vi "Scope_5782_PID_test.vi"() -> ()   [LabVIEW 2013]
uses:
  <vilib>/userdefined/High Color/nirio_resource_hc.ctl
  FPGA/DataMode.ctl
  <vilib>/Analysis/4window.llb/windowTd.ctl
  Host/Scope/controls/power_spectrum_unit.ctl
  Host/Scope5782/Scope/controls/5782_trigger_type.ctl
  Host/Scope/controls/Data_calc_mode.ctl
  Host/Scope/controls/Data_display_mode.ctl
  Host/Scope/controls/Graph_references.ctl
  Host/Scope/controls/graph_controls.ctl
  Host/Scope/controls/Channel_select.ctl
  Host/Scope5782/Config/FPGAref_5782.ctl
  Host/Scope/controls/ScopeMode.ctl
  <vilib>/FPGAPlugInAG/PXIe-7975R/niLvFpga_Open_PXIe-7975R.vi
  <vilib>/rvi/interface/common/dynamic/niFpgaDynamicAddResources.vi
  <vilib>/rvi/interface/common/niFpgaWaitOnOcc.vi
  <vilib>/Utility/error.llb/Error Cluster From Error Code.vi
  <vilib>/rvi/errors/niLvFpgaAdjustHostInterfaceError.vi
  <vilib>/FPGAPlugInAG/Dynamic/niLvFpga_Close_Dynamic.vi
  <vilib>/rvi/interface/nirviOpenFPGA/nirviOpenFPGA.xnode
  FPGA Bitfiles/mixer_FPGATarget2_FPGAmain5782PIDt_FQeTUQzgJng.lvbitx
  <vilib>/rvi/interface/nirviReadWriteControl/nirviReadWriteControl.xnode
  <vilib>/rvi/interface/nirviCloseFPGA/nirviCloseFPGA.xnode
  Host/Utilities/Ticker/Ticker.lvclass
  NiFpgaLv.dll
  <vilib>/rvi/interface/Simulation/niFpgaSimulationCallBeginRW.vi
  <vilib>/Analysis/NI_AALPro.lvlib
panel:
  in  "Kp":fxp<+/-,32,4>
  in  "Kd/T":fxp<+/-,32,4>
  in  "Ki*T":fxp<+/-,32,4>
  in  "Feedback":bool
  in  "b":fxp<+/-,16,2>
  in  "a":fxp<+/-,16,2>
  in  "Fequency [kHz]":dbl format="%#_8g"
  in  "#bins":i32=1 min=1 max=16
  in  "ch1 DC offset":i16 caption="DC offset\nChannel 1"
  in  "ch0 DC offset":i16 caption="DC offset\nChannel 0"
  in  "Output delay delta":dbl(slide) scale=0.0..6.0
  in  "Output delay":dbl(slide) scale=0.0..6.0
  in  "Chart length":i32=200000
  in  "Trigmode":enum32{"Triggered", "Continuous"}(radio)
  in  "Refence for phase":T1
  in  "Graph_refs":T2
  out "Lower chart":dbl[][](graph)
  out "Upper chart":dbl[][](graph)
  out "Lower graph":i16[][](graph)
  in  "Buffer":T4
  in  "Display":T5
  in  "Output mixer fequency [MHz]":dbl
  in  "Trigger":T6
  in  "Ch1 Q":bool
  in  "Ch1 I":bool
  in  "Ch0 Q":bool
  in  "Ch0 I":bool
  in  "Ch1":bool
  in  "Ch0":bool
  out "stop 2":bool
  in  "Zoom freq X":bool
  in  "Zoom freq Y":bool
  in  "Zoom time Y":bool
  in  "Zoom time X":bool
  in  "Unit":T7
  in  "Window":T8=1 items=["Rectangle"=0, "Hanning"=1, "Hamming"=2, "Blackman-Harris"=3, "Exact Blackman"=4, "Blackman"=5, "Flat Top"=6, "4 Term B-Harris "=7, "7 Term B-Harris"=8, "Low Sidelobe"=9, "Blackman Nuttall"=11, "Triangle"=30, "Bartlett-Hanning"=31, "Bohman"=32, "Parzen"=33, "Welch"=34, "Kaiser"=60, "Dolph-Chebyshev"=61, "Gaussian"=62]
  in  "Samples per 5782 record":i32
  in  "Phase offset (deg)":dbl
  in  "Fequency [MHz]":dbl format="%#_8g"
  in  "Mode":T9
  in  "Mixer freq [MHz]":dbl
  out "freqdata":cluster{"f0":dbl, "df":dbl, "magnitude":dbl[]}[](graph)
  out "Upper graph":i16[][](graph)
  in  "Rumode":bool
  in  "Singleshot":bool
  out "error IO":errorcluster
  in  "stop":bool
  in  "resource name":T10="RIO0"
  out "Clocking Option Configured?":bool
  out "Configured?":bool
  # "FPGA setup"
  # "ADU"
  # "ADU"
  # "Output delay"
  # "ns"
  # "Auto Zoom"
  # "Output delay delta"
  # "ps"
  # "5782"
  # "Amplitude modulation"
  # "Simulated data"
  # "FFT"
  # "Auto Zoom"
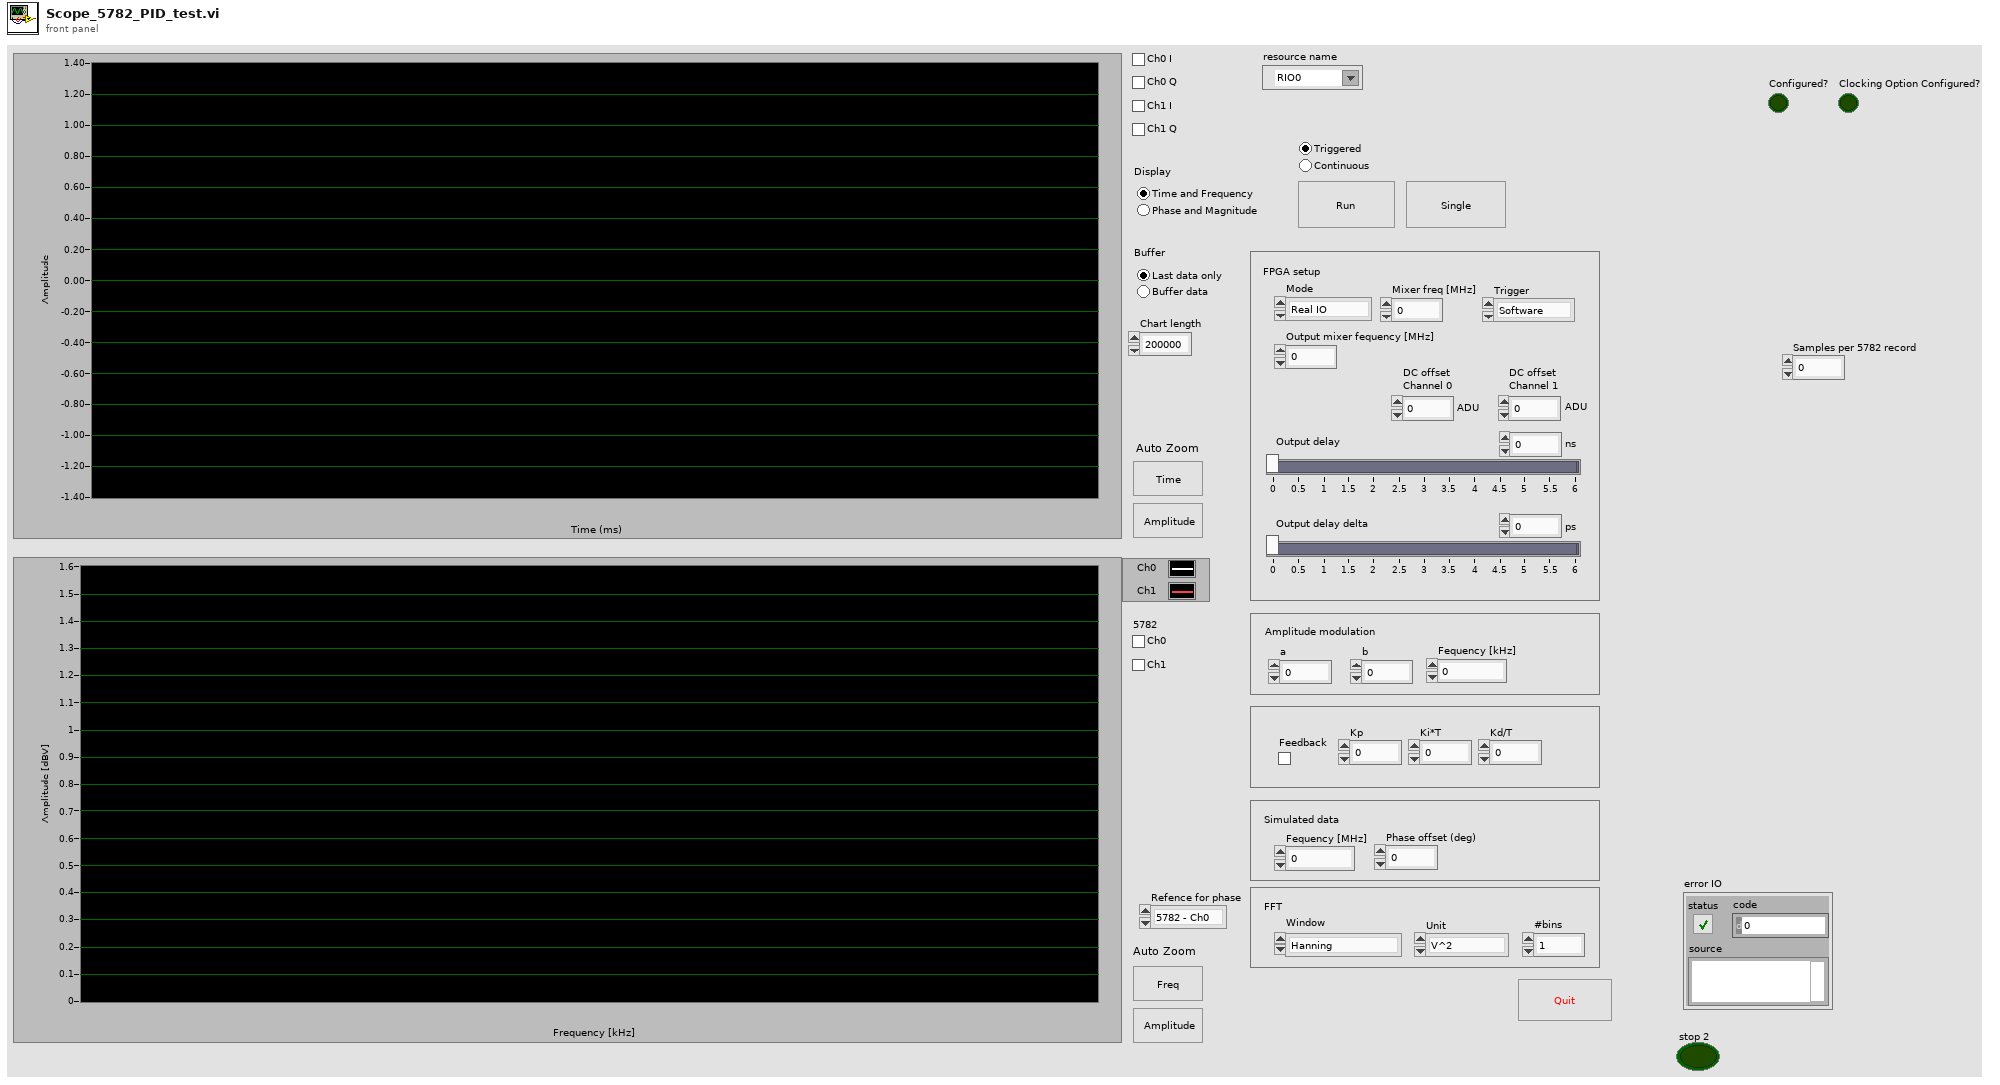
[diagram p1: front panel]
types:
  T1 = typedef "Channel_select.ctl" = enum16{"5782 - Ch0", "5782 - Ch1"}
  T2 = typedef "Graph_references.ctl" = cluster{"upper":T3, "lower":T3, "Freq graph":refnum<vi>}
  T3 = typedef "graph_controls.ctl" = cluster{"Graph":refnum<vi>, "Time btn":refnum<vi>, "Amplitude btn":refnum<vi>, "Chart":refnum<vi>}
  T4 = typedef "Data_display_mode.ctl" = enum32{"Last data only", "Buffer data"}
  T5 = typedef "Data_calc_mode.ctl" = enum32{"Time and Frequency", "Phase and Magnitude"}
  T6 = typedef "5782_trigger_type.ctl" = enum16{"Software", "Trigger input"}
  T7 = typedef "power_spectrum_unit.ctl" = enum16{"V^2", "V", "dBV"}
  T8 = typedef "NI_AALPro.lvlib/windowTd.ctl" = u32
  T9 = typedef "DataMode.ctl" = enum16{"Real IO", "Simulated"}
  T10 = typedef "nirio_resource_hc.ctl" = tag
  T11 = typedef "FPGAref_5782.ctl" = refnum<k20>
  T12 = enum8{"Internal Clock PLL Off", "Internal Clock PLL On (REF IN)", "External Clock (CLK_IN)", "Internal Clock PLL On (IoModSyncClk)"}
  T13 = typedef "scope_params_5782.ctl" = cluster{"scope mode":T14, "ticker":refnum<class "Ticker.lvclass">, "samples per record":i32, "FPGA ref":T11, "data mode":T9, "5782 Trigger":T6, "Chart length":i32}
  T14 = typedef "ScopeMode.ctl" = enum16{"Stopped", "Single", "Running", "Continuous"}
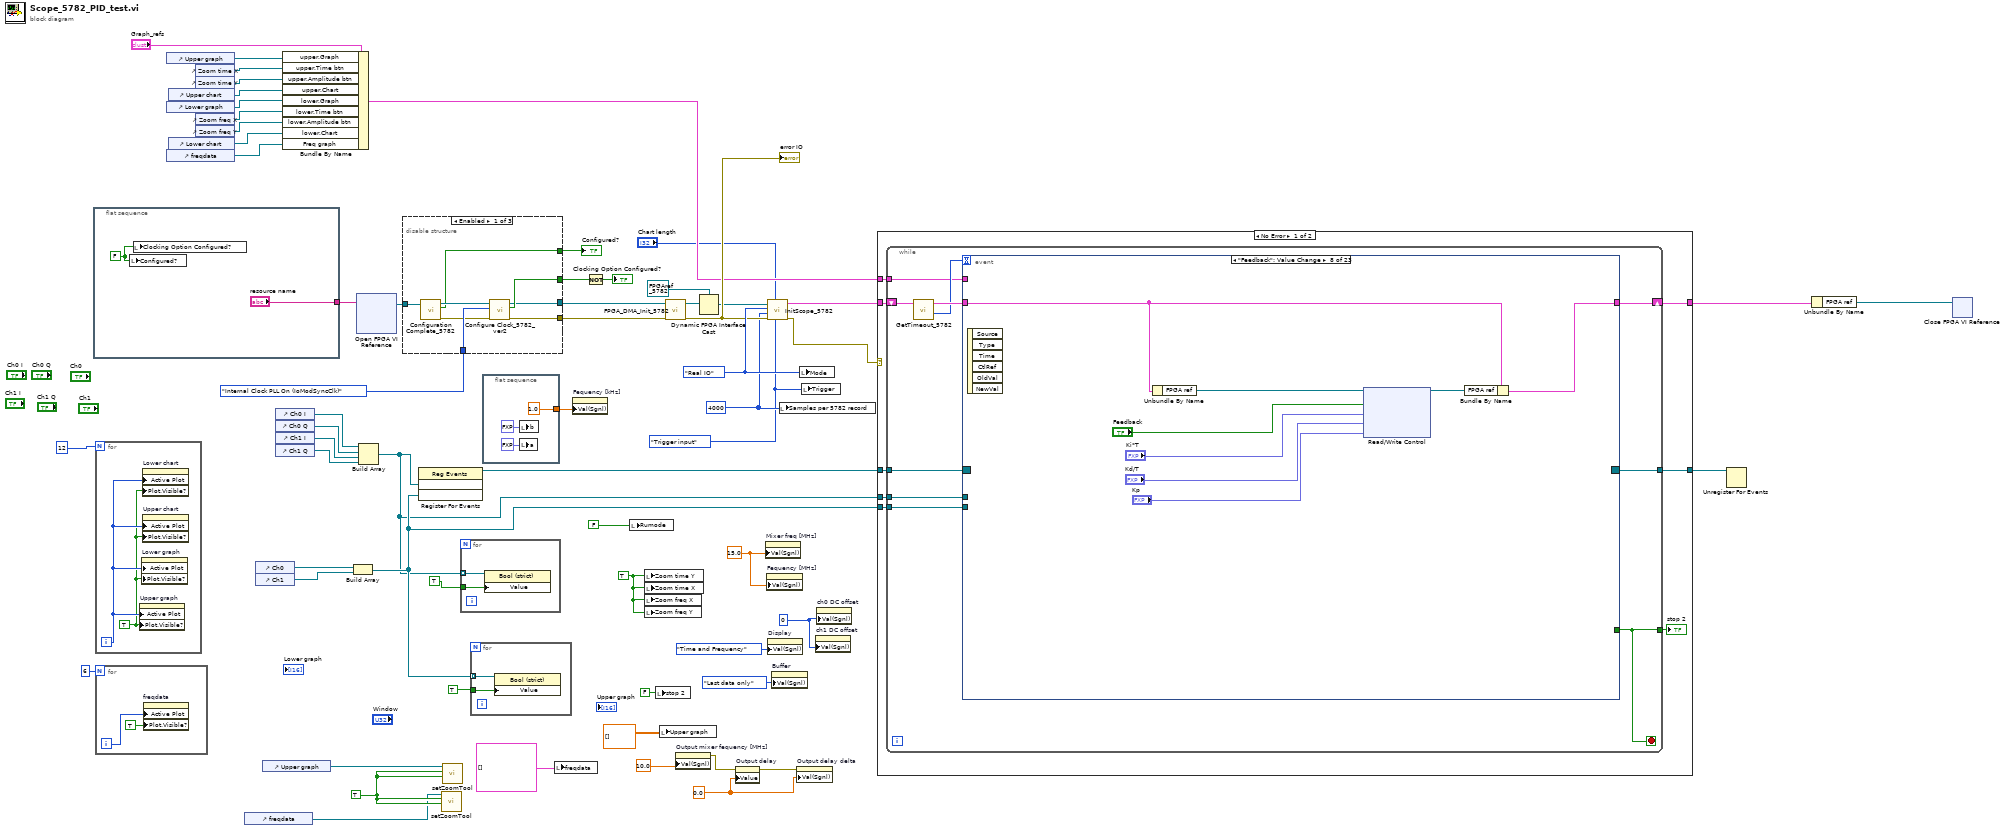
[diagram p0: block diagram]
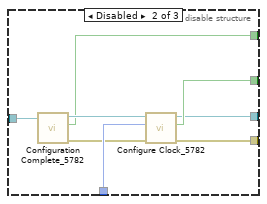
[diagram p2: hidden frame]
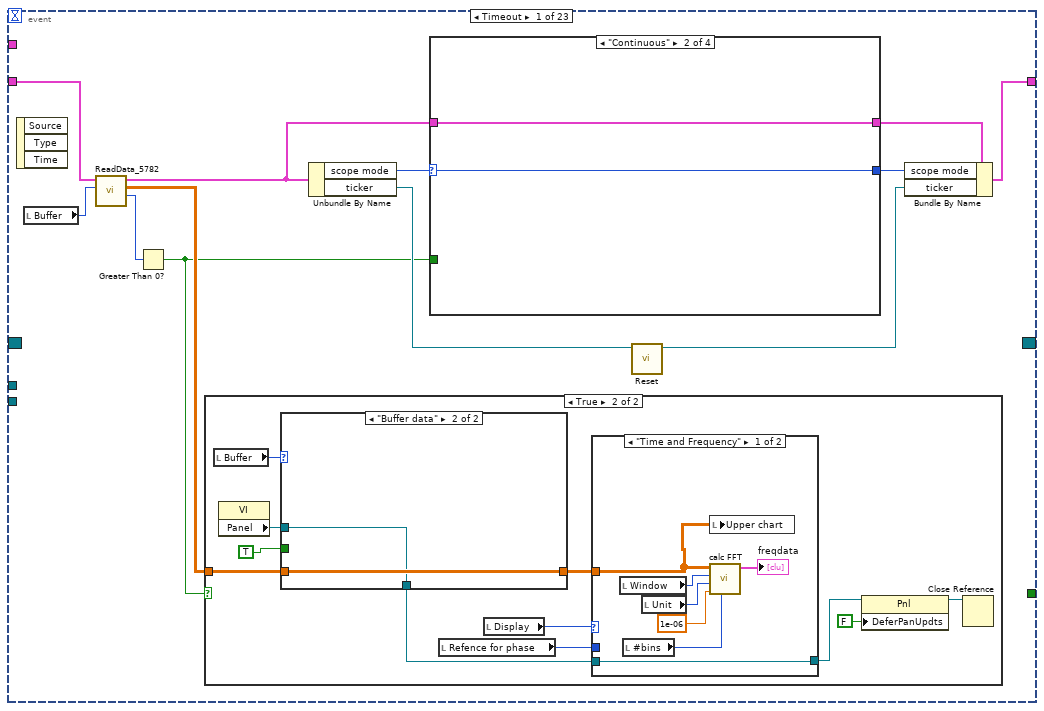
[diagram p4: hidden frame]
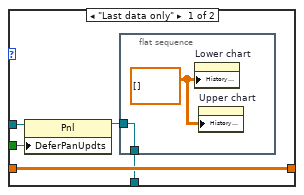
[diagram p6: hidden frame]
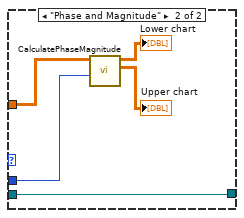
[diagram p7: hidden frame]
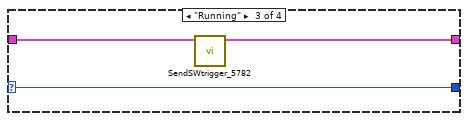
[diagram p9: hidden frame]
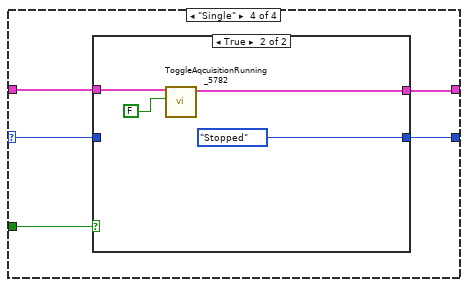
[diagram p10: hidden frame]
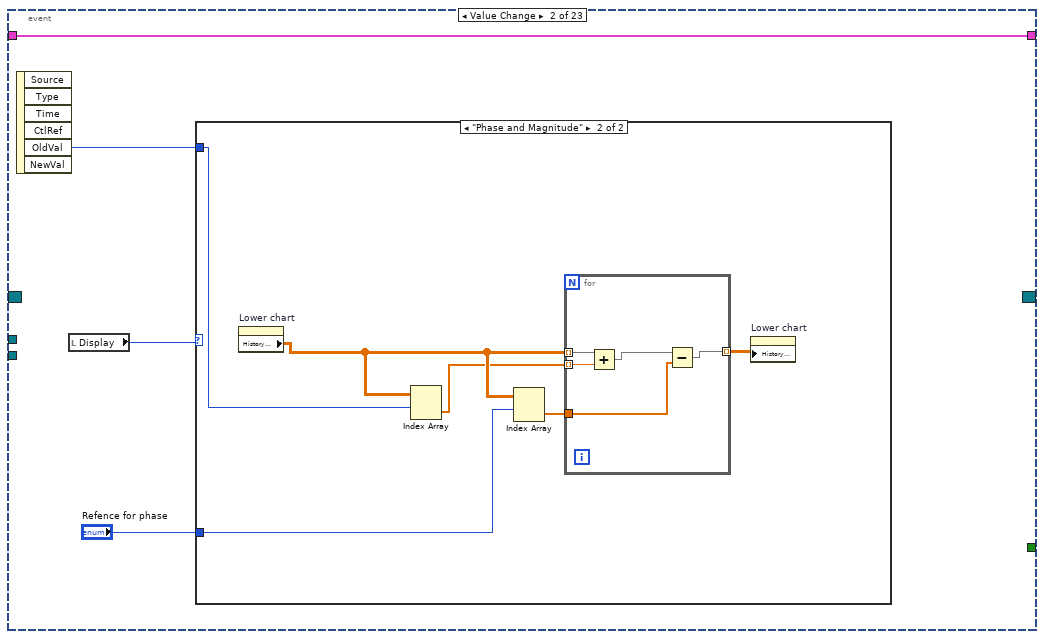
[diagram p12: hidden frame]
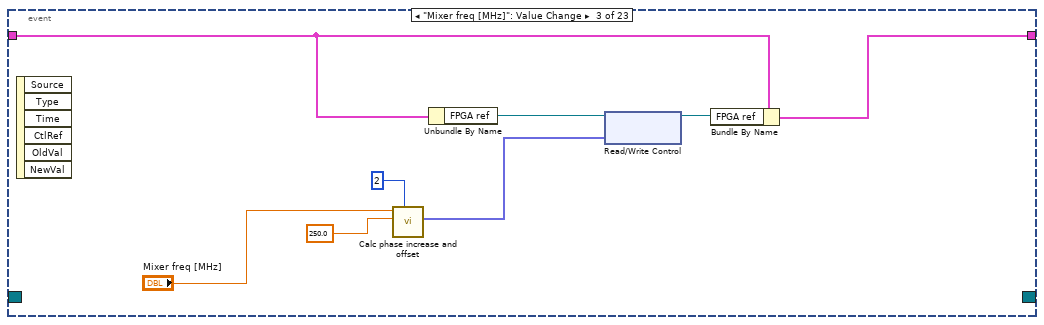
[diagram p14: hidden frame]
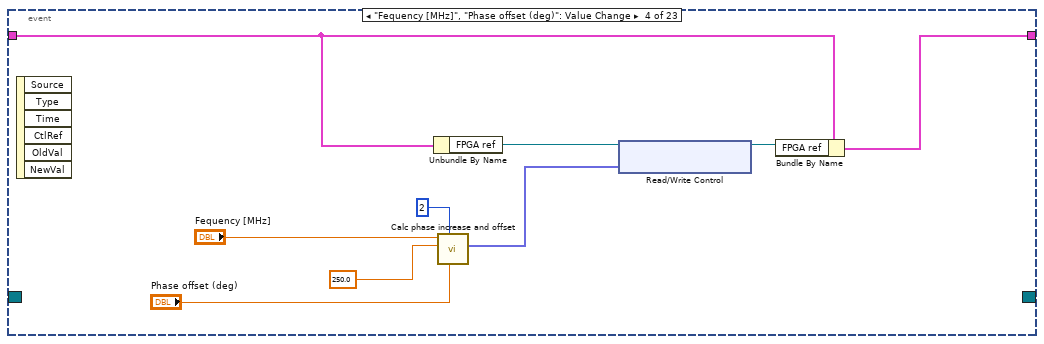
[diagram p15: hidden frame]
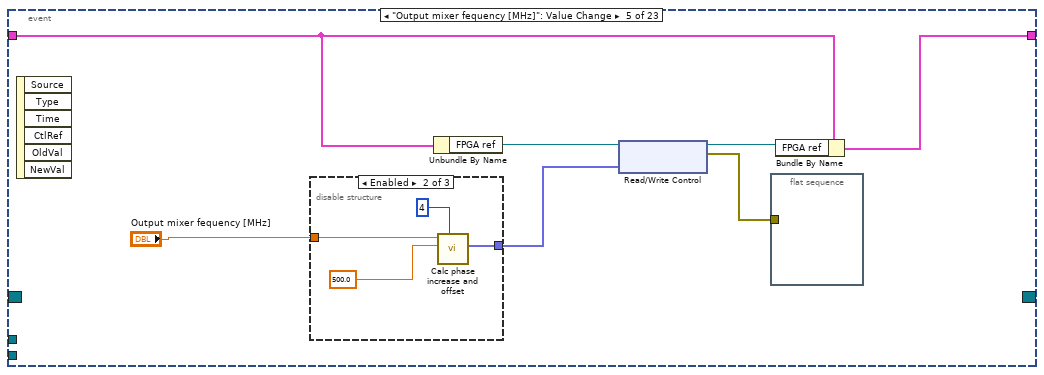
[diagram p16: hidden frame]
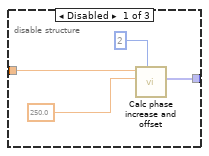
[diagram p17: hidden frame]
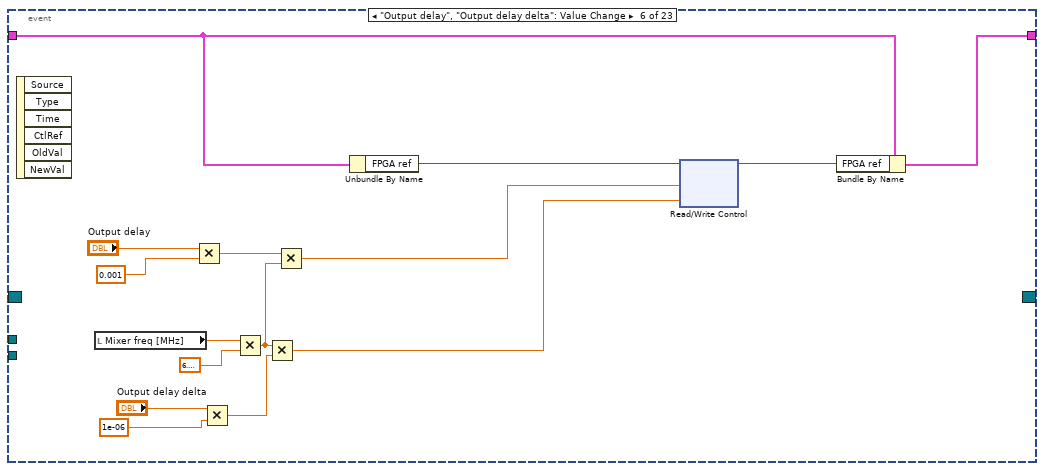
[diagram p19: hidden frame]
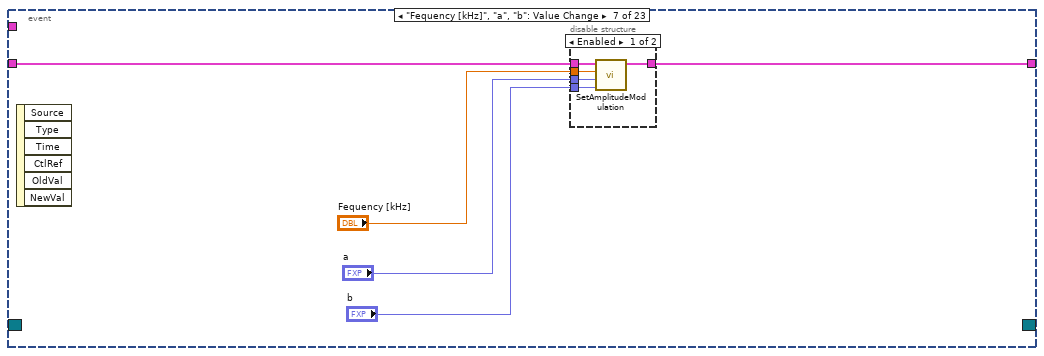
[diagram p20: hidden frame]
diagram:
  w6 = i16 0 ("Value (Signaling)")
  w7 = 0.0 ("Value (Signaling)")
  w31 = 5782_trigger_type."Trigger input" ("Trigger")
  w37 = TRUE ("Zoom  X")
  w47 = TRUE ("Rumode")
  w46 = DataMode."Real IO" ("Mode")
  w33 = 4000 ("Samples to aqcuire")
  w58 = 15.0 ("Mixer requency [MHz]")
  n1 = flat-sequence {
    tunnel: ["resource name"] -> w48
    frame #0 {
      w63 = FALSE ("Trigger Acquisition")
      n2 = local write "Configured?"(w63) -> ()
      n3 = local write "Clocking Option Configured?"(w63) -> ()
    }
  }
  n4 = for {
    N: 12 -> [_]
    i -> [w66]
    w65 = TRUE ("Plot.Visible")
    n5 = property on="Upper graph" class="WFGraph (strict)"("Active Plot"=w66, "Plot.Visible?"=w65) -> ()  [unwired: 2 in, 2 out]
    n6 = property on="Lower graph" class="WFGraph (strict)"("Active Plot"=w66, "Plot.Visible?"=w65) -> ()  [unwired: 2 in, 2 out]
    n7 = property on="Lower chart" class="WFChart (strict)"("Active Plot"=w66, "Plot.Visible?"=w65) -> ()  [unwired: 2 in, 2 out]
    n8 = property on="Upper chart" class="WFChart (strict)"("Active Plot"=w66, "Plot.Visible?"=w65) -> ()  [unwired: 2 in, 2 out]
  }
  n9 = for {
    N: 6 -> [_]
    i -> [w67]
    n10 = property on="freqdata" class="WFGraph (strict)"("Active Plot"=w67, "Plot.Visible?"=TRUE ("Plot.Visible")) -> ()  [unwired: 2 in, 2 out]
  }
  n11 = control-ref of="Upper graph"() -> (w28:refnum<vi>)
  n12 = control-ref of="Lower graph"() -> (w24:refnum<vi>)
  n13 = control-ref of="freqdata"() -> (w20:refnum<vi>)
  n14 = control-ref of="Upper chart"() -> (w25:refnum<vi>)
  n15 = control-ref of="Lower chart"() -> (w21:refnum<vi>)
  n16 = control-ref of="Zoom time X"() -> (w27:refnum<vi>)
  n17 = control-ref of="Zoom time Y"() -> (w26:refnum<vi>)
  n18 = control-ref of="Zoom freq X"() -> (w23:refnum<vi>)
  n19 = control-ref of="Zoom freq Y"() -> (w22:refnum<vi>)
  n20 = control-ref of="freqdata"() -> (w35:refnum<vi>)
  n21 = control-ref of="Ch0"() -> (w43:refnum<vi>)
  n22 = control-ref of="Ch1"() -> (w44:refnum<vi>)
  n23 = control-ref of="Upper graph"() -> (w36:refnum<vi>)
  n24 = control-ref of="Ch0 I"() -> (w39:refnum<vi>)
  n25 = control-ref of="Ch0 Q"() -> (w40:refnum<vi>)
  n26 = control-ref of="Ch1 I"() -> (w41:refnum<vi>)
  n27 = control-ref of="Ch1 Q"() -> (w42:refnum<vi>)
  n28 = Bundle By Name(cluster="Graph_refs", "upper.Graph"=w28, "upper.Time btn"=w27, "upper.Amplitude btn"=w26, "upper.Chart"=w25, "lower.Graph"=w24, "lower.Time btn"=w23, "lower.Amplitude btn"=w22, "lower.Chart"=w21, "Freq graph"=w20) -> (w19:T2)
  n29 = Build Array(w43, w44) -> (w50:refnum<vi>[])
  n30 = xnode "Open FPGA VI Reference"("resource name"=w48) -> ("FPGA VI Reference Out"=w12:refnum<k20>)  [unwired: 1 in, 1 out]
  n31 = Build Array(w39, w40, w41, w42) -> (w38:refnum<vi>[])
  n32 = disable-structure shown="Enabled" {
    disable-tunnel: [w76 w84 _] -> w14
    disable-tunnel: T12."Internal Clock PLL On (IoModSyncClk)" ("Clock Source") -> [w75 w83 _]
    disable-tunnel: [w73 w81 _] -> w13
    disable-tunnel: [w71 w78 w85] -> w5
    disable-tunnel: w12 -> [w69 w80 w85]
    disable-tunnel: [w70 w77 _] -> w10
    frame Enabled {
      n33 = call "Configuration Complete_5782.vi"("FPGA VI Reference in"=w69) -> ("error out"=w74:errorcluster, "Configured?"=w70:bool, "FPGA VI Reference out"=w72:refnum<k20>)  [unwired: 8 in]
      n34 = call "Configure Clock_5782_ver2.vi"("error in"=w74, "Clock Source"=w75, "FPGA VI Reference"=w72) -> ("error out"=w73:errorcluster, "Configuration Error"=w76:bool, "FPGA VI Reference out"=w71:refnum<k20>)  [unwired: 6 in]
    }
    frame Disabled {
      n35 = call "Configuration Complete_5782.vi"("FPGA VI Reference in"=w80) -> ("error out"=w82:errorcluster, "Configured?"=w77:bool, "FPGA VI Reference out"=w79:refnum<k20>)  [unwired: 8 in]
      n36 = call "Configure Clock_5782.vi"("error in"=w82, "Clock Source"=w83, "FPGA VI Reference in"=w79) -> ("error out"=w81:errorcluster, "Configuration Error"=w84:bool, "FPGA VI Reference Out"=w78:T11)  [unwired: 6 in]
    }
    frame Disabled {
    }
  }
  "Configured?" <- w10
  n37 = register-events(w38, w50) -> (reference out=w54:refnum<event-registration>)  [unwired: 2 in, 1 out]
  n38 = call "setZoomTool.vi"("Zoom Y"=w37, "Zoom  X"=w37, "reference"=w35) -> ()  [unwired: 9 in]
  n39 = call "setZoomTool.vi"("Zoom Y"=w37, "Zoom  X"=w37, "reference"=w36) -> ()  [unwired: 9 in]
  n40 = for {
    tunnel: w38 -> [w87] mode=indexing
    tunnel: TRUE ("Rumode") -> [w86]
    n41 = property class="Bool (strict)"(reference=w87, "Value"=w86) -> ()  [unwired: 1 in, 2 out]
  }
  n42 = for {
    tunnel: w50 -> [w89] mode=indexing
    tunnel: TRUE ("Rumode") -> [w88]
    n43 = property class="Bool (strict)"(reference=w89, "Value"=w88) -> ()  [unwired: 1 in, 2 out]
  }
  n44 = flat-sequence {
    tunnel: [1.0 ("Value (Signaling)")] -> w4
    frame #0 {
      n45 = local write "b"(fxp<+/-,16,2> 0.0 ("b")) -> ()
      n46 = local write "a"(fxp<+/-,16,2> 1.0 ("a")) -> ()
    }
  }
  n47 = local write "freqdata"(cluster{"f0":dbl, "df":dbl, "magnitude":dbl[]}[] [] ("freqdata")) -> ()
  n48 = property on="Fequency [kHz]" class="DigNum (strict)"("Val(Sgnl)"=w4) -> ()  [unwired: 2 in, 2 out]
  n49 = Not(x=w14) -> (.not. x?=→"Clocking Option Configured?":bool)
  n50 = local write "Rumode"(FALSE ("Rumode")) -> ()
  n51 = local write "Zoom time Y"(w47) -> ()
  n52 = local write "Zoom time X"(w47) -> ()
  n53 = local write "Zoom freq X"(w47) -> ()
  n54 = local write "Zoom freq Y"(w47) -> ()
  n55 = local write "stop 2"(FALSE ("stop 2")) -> ()
  n56 = local write "Upper graph"(dbl[][] [] ("Timedata")) -> ()
  n57 = call "FPGA_DMA_Init_5782.vi"("error in (no error)"=w13, "FPGA VI Reference"=w5) -> ("error out"=w34:errorcluster, "FPGA VI Out"=w3:refnum<k20>)  [unwired: 7 in, 1 out]
  "error IO" <- w34
  n58 = property on="Output mixer fequency [MHz]" class="DigNum (strict)"("Val(Sgnl)"=10.0 ("Mixer requency [MHz]")) -> (error out=w8:errorcluster)  [unwired: 2 in, 1 out]
  n59 = Dynamic FPGA Interface Cast(Session In=T11 refnum ("FPGA ref"), Type=w3) -> (Session Out=w2:T11)
  n60 = property on="Output delay" class="Slide (strict)"(error in=w8, "Value"=w7) -> (error out=w9:errorcluster)  [unwired: 1 in, 1 out]
  n61 = property on="Mixer freq [MHz]" class="DigNum (strict)"("Val(Sgnl)"=w58) -> ()  [unwired: 2 in, 2 out]
  n62 = property on="Fequency [MHz]" class="DigNum (strict)"("Val(Sgnl)"=w58) -> ()  [unwired: 2 in, 2 out]
  n63 = call "InitScope_5782.vi"("Trigger"=w31, "Chart length"="Chart length", "error in"=w34, "Samples Per Trigger"=w33, "data mode"=w46, "FPGA ref"=w2) -> ("error out"=w18:errorcluster, "scope params"=w62:T13)  [unwired: 4 in]
  n64 = property on="Display" class="RadioBtnsControl (strict)"("Val(Sgnl)"=Data_calc_mode."Time and Frequency" ("Value (Signaling)")) -> ()  [unwired: 2 in, 2 out]
  n65 = property on="Buffer" class="RadioBtnsControl (strict)"("Val(Sgnl)"=enum32{"Last data only", "Buffer data"}."Last data only" ("Value (Signaling)")) -> ()  [unwired: 2 in, 2 out]
  n66 = local write "Samples per 5782 record"(w33) -> ()
  n67 = property on="Output delay delta" class="Slide (strict)"(error in=w9, "Val(Sgnl)"=w7) -> ()  [unwired: 1 in, 2 out]
  n68 = local write "Mode"(w46) -> ()
  n69 = local write "Trigger"(w31) -> ()
  n70 = property on="ch1 DC offset" class="DigNum (strict)"("Val(Sgnl)"=w6) -> ()  [unwired: 2 in, 2 out]
  n71 = property on="ch0 DC offset" class="DigNum (strict)"("Val(Sgnl)"=w6) -> ()  [unwired: 2 in, 2 out]
  n72 = case shown="No Error" w18 {
    tunnel: w62 -> [w100 w364]
    tunnel: [w99 w364] -> w32
    tunnel: w54 -> [w98 w363]
    tunnel: [w97 w363] -> w53
    tunnel: w38 -> [w96 _]
    tunnel: w50 -> [w95 _]
    tunnel: w19 -> [w93 _]
    frame No Error {
      n73 = while {
        shift-right: [w110] -> w99
        shift-left: w100 -> [w109]
        tunnel: w98 -> [w106]
        tunnel: [w105] -> w97
        tunnel: w96 -> [w104]
        tunnel: w95 -> [w103]
        tunnel: [w102] -> w94
        tunnel: w93 -> [w101]
        stop <- w102 stop-if-true
        n74 = call "GetTimeout_5782.vi"("scope in"=w109) -> ("Time left"=w107:i32, "scope out"=w108:T13)  [unwired: 9 in]
        n75 = event shown="[7] \"Feedback\": Value Change" {
          selector: w106 -> [_ _ _ _ _ _ _ _ _ _ _ _ _ _ _ _ _ _ _ _ _ _ _]
          dyn-events: [_ _ _ _ _ _ _ _ _ _ _ _ _ _ _ _ _ _ _ _ _ _ _] -> w105
          timeout: w107 -> [_ _ _ _ _ _ _ _ _ _ _ _ _ _ _ _ _ _ _ _ _ _ _]
          tunnel: [_ _ _ _ _ _ _ _ _ _ _ _ _ _ _ _ _ "stop" _ _ _ _ _] -> w102
          tunnel: w108 -> [w117 w176 w194 w200 w209 w230 w239 w251 w258 w265 w271 w275 w278 w288 w296 w321 w326 w327 w334 w344 w349 w355 w362]
          tunnel: [w120 w176 w192 w199 w208 w229 w238 w250 w257 w264 w270 w274 w277 w285 w293 w321 w326 w327 w334 w344 w349 w355 w362] -> w110
          tunnel: w104 -> [_ _ _ _ _ _ _ _ _ _ _ _ _ _ _ w320 _ _ _ _ _ _ _]
          tunnel: w103 -> [_ _ _ _ _ _ _ _ _ _ _ _ _ _ _ _ w324 _ _ _ _ _ _]
          tunnel: w101 -> [_ _ _ _ _ _ _ _ _ _ _ _ _ _ _ _ _ _ _ _ _ _ w359]
          event Timeout {
            n76 = event-data() -> ()  [unwired: 1 in, 3 out]
            n77 = local read "Buffer"() -> (w111:T4)
            n78 = call "ReadData_5782.vi"("Buffer mode"=w111, "scope params"=w117) -> ("Num elements"=w113:i32, "data"=w114:dbl[][], "scope params out"=w116:T13)  [unwired: 7 in]
            n79 = Greater Than 0?(x=w113) -> (x > 0?=w112:bool)
            n80 = case shown="True" w112 {
              tunnel: w114 -> [_ w130]
              frame False {
              }
              frame True {
                n81 = local read "Buffer"() -> (w132:T4)
                n82 = property class="VI"() -> ("Panel"=w125:refnum<vi>)  [unwired: 2 in, 2 out]
                n83 = case shown="\"Buffer data\"" w132 {
                  tunnel: w130 -> [w138 w142]
                  tunnel: [w138 w142] -> w131
                  tunnel: w125 -> [w137 w141]
                  tunnel: TRUE ("Defer Panel Updates") -> [w135 _]
                  tunnel: [w134 w141] -> w123
                  frame "Last data only" {
                    n84 = property class="Pnl"(reference=w137, "DeferPanUpdts"=w135) -> (reference out=w136:refnum<vi>)  [unwired: 1 in, 1 out]
                    n85 = flat-sequence {
                      tunnel: w136 -> [w139]
                      tunnel: [w139] -> w134
                      frame #0 {
                        w140 = dbl[][] [] ("History Data")
                        n86 = property on="Lower chart" class="WFChart (strict)"("History Data"=w140) -> ()  [unwired: 2 in, 2 out]
                        n87 = property on="Upper chart" class="WFChart (strict)"("History Data"=w140) -> ()  [unwired: 2 in, 2 out]
                      }
                    }
                  }
                  frame "Buffer data" {
                  }
                }
                n88 = local read "Refence for phase"() -> (w129:T1)
                n89 = local read "Display"() -> (w133:T5)
                n90 = case shown="\"Time and Frequency\"" w133 {
                  tunnel: w131 -> [w145 w154]
                  tunnel: w129 -> [_ w151]
                  tunnel: [w144 w150] -> w127
                  tunnel: w123 -> [w144 w150]
                  frame "Time and Frequency" {
                    n91 = local read "Window"() -> (w146:T8)
                    n92 = local read "#bins"() -> (w143:i32)
                    n93 = local read "Unit"() -> (w147:T7)
                    n94 = local write "Upper chart"(w145) -> ()
                    n95 = call "calc FFT.vi"("#bins"=w143, "dt"=1e-06, "Unit"=w147, "Window"=w146, "data"=w145) -> ("Power Spectrum / PSD"=→"freqdata":cluster{"f0":dbl, "df":dbl, "magnitude":dbl[]}[])  [unwired: 6 in]
                  }
                  frame "Phase and Magnitude" {
                    n96 = call "CalculatePhaseMagnitude.vi"("phase reference channel"=w151, "data"=w154) -> ("Magnitude"=→"Upper chart":dbl[][], "Phase"=→"Lower chart":dbl[][])  [unwired: 8 in]
                  }
                }
                n97 = property class="Pnl"(reference=w127, "DeferPanUpdts"=FALSE ("Defer Panel Updates")) -> (reference out=w126:refnum<vi>)  [unwired: 1 in, 1 out]
                n98 = Close Reference(reference=w126) -> ()  [unwired: 1 in, 1 out]
              }
            }
            n99 = Unbundle By Name(w116) -> ("scope mode"=w119:T14, "ticker"=w122:refnum<class "Ticker.lvclass">)
            n100 = case shown="\"Continuous\"" w119 {
              selector: w119 -> [w156 w158 w161 w162]
              tunnel: [w156 w158 w161 w166] -> w118
              tunnel: w116 -> [w155 w157 w160 w164]
              tunnel: [w155 w157 w159 w163] -> w115
              tunnel: w112 -> [_ _ _ w165]
              frame "Stopped" {
              }
              frame "Continuous" {
              }
              frame "Running" {
                n101 = call "SendSWtrigger_5782.vi"("scope in"=w160) -> ("scope out"=w159:T13)  [unwired: 9 in, 1 out]
              }
              frame "Single" {
                n102 = case shown="True" w165 {
                  tunnel: [w167 ScopeMode."Stopped" ("scope mode")] -> w166
                  tunnel: w164 -> [w168 w171]
                  tunnel: [w168 w170] -> w163
                  tunnel: w162 -> [w167 _]
                  frame False {
                  }
                  frame True {
                    n103 = call "ToggleAqcuisitionRunning_5782.vi"("Acquisition running"=FALSE, "scope in"=w171) -> ("scope out"=w170:T13)  [unwired: 8 in, 1 out]
                  }
                }
              }
            }
            n104 = call "Reset.vi"("Ticker in"=w122) -> ("Ticker out"=w121:refnum<class "Ticker.lvclass">)  [unwired: 9 in, 1 out]
            n105 = Bundle By Name(cluster=w115, "scope mode"=w118, "ticker"=w121) -> (w120:T13)
          }
          event Value Change {
            n106 = event-data() -> ("OldVal"=w173:T1)  [unwired: 1 in, 5 out]
            n107 = local read "Display"() -> (w174:T5)
            n108 = case shown="\"Phase and Magnitude\"" w174 {
              tunnel: "Refence for phase" -> [_ w181]
              tunnel: w173 -> [_ w179]
              frame "Time and Frequency", Default {
              }
              frame "Phase and Magnitude" {
                n109 = property on="Lower chart" class="WFChart (strict)"() -> ("History Data"=w180:dbl[][])  [unwired: 2 in, 2 out]
                n110 = Index Array(array=w180, index (row)=w179) -> (element=w178:dbl[])  [unwired: 1 in]
                n111 = Index Array(array=w180, index (row)=w181) -> (element=w182:dbl[])  [unwired: 1 in]
                n112 = for {
                  tunnel: w180 -> [w185] mode=indexing
                  tunnel: w182 -> [w187]
                  tunnel: [w186] -> w177 mode=indexing
                  tunnel: w178 -> [w184] mode=indexing
                  n113 = Add(x=w185, y=w184) -> (x+y=w183:dbl[])
                  n114 = Subtract(x=w183, y=w187) -> (x-y=w186:dbl[])
                }
                n115 = property on="Lower chart" class="WFChart (strict)"("History Data"=w177) -> ()  [unwired: 2 in, 2 out]
              }
            }
          }
          event "Mixer freq [MHz]": Value Change {
            n116 = event-data() -> ()  [unwired: 1 in, 6 out]
            n117 = call "Calc phase increase and offset.vi"("# of DDS"=2, "fclk (MHz)"=250.0 ("fclk (800MHz)"), "f_generated (MHz)"="Mixer freq [MHz]") -> ("Phase out"=w188:fxp<+,64,64>[])  [unwired: 6 in, 2 out]
            n118 = Unbundle By Name(w194) -> ("FPGA ref"=w195:T11)
            n119 = xnode "Read/Write Control"("FPGA VI Reference In"=w195, "Phase 5782"=w188) -> ("FPGA VI Reference Out"=w193:T11)  [unwired: 1 in, 1 out]
            n120 = Bundle By Name(cluster=w194, "FPGA ref"=w193) -> (w192:T13)
          }
          event "Fequency [MHz]", "Phase offset (deg)": Value Change {
            n121 = event-data() -> ()  [unwired: 1 in, 6 out]
            n122 = Unbundle By Name(w200) -> ("FPGA ref"=w202:T11)
            n123 = call "Calc phase increase and offset.vi"("Phase offset (deg)"="Phase offset (deg)", "# of DDS"=2, "fclk (MHz)"=250.0 ("fclk (800MHz)"), "f_generated (MHz)"="Fequency [MHz]") -> ("Phase out"=w196:fxp<+,64,64>[])  [unwired: 5 in, 2 out]
            n124 = xnode "Read/Write Control"("FPGA VI Reference In"=w202, "Simulated phase 5782"=w196) -> ("FPGA VI Reference Out"=w201:T11)  [unwired: 1 in, 1 out]
            n125 = Bundle By Name(cluster=w200, "FPGA ref"=w201) -> (w199:T13)
          }
          event "Output mixer fequency [MHz]": Value Change {
            n126 = event-data() -> ()  [unwired: 1 in, 6 out]
            n127 = disable-structure shown="Enabled" {
              disable-tunnel: [w213 w217 _] -> w205
              disable-tunnel: "Output mixer fequency [MHz]" -> [w212 w216 _]
              frame Disabled {
                n128 = call "Calc phase increase and offset.vi"("# of DDS"=2, "fclk (MHz)"=250.0 ("fclk (800MHz)"), "f_generated (MHz)"=w212) -> ("Phase out"=w213:fxp<+,64,64>[])  [unwired: 6 in, 2 out]
              }
              frame Enabled {
                n129 = call "Calc phase increase and offset.vi"("# of DDS"=4, "fclk (MHz)"=500.0 ("fclk (800MHz)"), "f_generated (MHz)"=w216) -> ("Phase out"=w217:fxp<+,64,64>[])  [unwired: 6 in, 2 out]
              }
              frame Disabled {
              }
            }
            n130 = Unbundle By Name(w209) -> ("FPGA ref"=w211:T11)
            n131 = xnode "Read/Write Control"("FPGA VI Reference In"=w211, "Phase output"=w205) -> ("FPGA VI Reference Out"=w210:T11, "error out"=w206:errorcluster)  [unwired: 1 in]
            n132 = flat-sequence {
              tunnel: w206 -> [_]
              frame #0 {
              }
            }
            n133 = Bundle By Name(cluster=w209, "FPGA ref"=w210) -> (w208:T13)
          }
          event "Output delay", "Output delay delta": Value Change {
            n134 = event-data() -> ()  [unwired: 1 in, 6 out]
            n135 = local read "Mixer freq [MHz]"() -> (w224:dbl)
            n136 = Multiply(x="Output delay", y=0.001) -> (x*y=w225:dbl)
            n137 = Multiply(x="Output delay delta", y=1e-06) -> (x*y=w227:dbl)
            n138 = Multiply(x=w224, y=6.283185307179586) -> (x*y=w220:dbl)
            n139 = Multiply(x=w220, y=w227) -> (x*y=w221:dbl)
            n140 = Multiply(x=w225, y=w220) -> (x*y=w222:dbl)
            n141 = Unbundle By Name(w230) -> ("FPGA ref"=w234:T11)
            n142 = xnode "Read/Write Control"("FPGA VI Reference In"=w234, "Fi_start"=w222, "Fi_delta"=w221) -> ("FPGA VI Reference Out"=w233:T11)  [unwired: 1 in, 1 out]
            n143 = Bundle By Name(cluster=w230, "FPGA ref"=w233) -> (w229:T13)
          }
          event "Fequency [kHz]", "a", "b": Value Change {
            n144 = event-data() -> ()  [unwired: 1 in, 6 out]
            n145 = disable-structure shown="Enabled" {
              disable-tunnel: w239 -> [w244 w245]
              disable-tunnel: [w243 w245] -> w238
              disable-tunnel: "Fequency [kHz]" -> [w242 _]
              disable-tunnel: "a" -> [w241 _]
              disable-tunnel: "b" -> [w240 _]
              frame Enabled {
                n146 = call "SetAmplitudeModulation.vi"("b_am"=w240, "a_am"=w241, "Am freq [kHz]"=w242, "scope in"=w244) -> ("scope out"=w243:T13)  [unwired: 7 in]
              }
              frame Disabled {
              }
            }
          }
          event "Feedback": Value Change {
            n147 = event-data() -> ()  [unwired: 1 in, 6 out]
            n148 = Unbundle By Name(w251) -> ("FPGA ref"=w253:T11)
            n149 = xnode "Read/Write Control"("FPGA VI Reference In"=w253, "feedback enable"="Feedback", "Ki*Tau"="Ki*T", "Kd/Tau"="Kd/T", "Kp"="Kp") -> ("FPGA VI Reference Out"=w252:T11)  [unwired: 1 in, 1 out]
            n150 = Bundle By Name(cluster=w251, "FPGA ref"=w252) -> (w250:T13)
          }
          event "ch0 DC offset": Value Change {
            n151 = event-data() -> ()  [unwired: 1 in, 6 out]
            n152 = Unbundle By Name(w258) -> ("FPGA ref"=w260:T11)
            n153 = Integer to Fixed-Point Cast(fixed-point type=fxp<+/-,16,16> 0.0 ("y"), integer="ch0 DC offset") -> (fixed-point=w255:fxp<+/-,16,16>)
            n154 = xnode "Read/Write Control"("FPGA VI Reference In"=w260, "DC offset chan 0"=w255) -> ("FPGA VI Reference Out"=w259:T11)  [unwired: 1 in, 1 out]
            n155 = Bundle By Name(cluster=w258, "FPGA ref"=w259) -> (w257:T13)
          }
          event "ch1 DC offset": Value Change {
            n156 = event-data() -> ()  [unwired: 1 in, 6 out]
            n157 = Unbundle By Name(w265) -> ("FPGA ref"=w267:T11)
            n158 = Integer to Fixed-Point Cast(fixed-point type=fxp<+/-,16,16> 0.0 ("y"), integer="ch1 DC offset") -> (fixed-point=w262:fxp<+/-,16,16>)
            n159 = xnode "Read/Write Control"("FPGA VI Reference In"=w267, "DC offset chan 1"=w262) -> ("FPGA VI Reference Out"=w266:T11)  [unwired: 1 in, 1 out]
            n160 = Bundle By Name(cluster=w265, "FPGA ref"=w266) -> (w264:T13)
          }
          event Value Change {
            n161 = event-data() -> ()  [unwired: 1 in, 6 out]
            n162 = Unbundle By Name(w271) -> ("FPGA ref"=w273:T11)
            n163 = property on="Rumode" class="Bool (strict)"("Val(Sgnl)"=FALSE ("Value (Signaling)")) -> ()  [unwired: 2 in, 2 out]
            n164 = xnode "Read/Write Control"("FPGA VI Reference In"=w273, "Mode"="Mode") -> ("FPGA VI Reference Out"=w272:T11)  [unwired: 1 in, 1 out]
            n165 = Bundle By Name(cluster=w271, "FPGA ref"=w272, "data mode"="Mode") -> (w270:T13)
          }
          event Value Change {
            n166 = event-data() -> ()  [unwired: 1 in, 6 out]
            n167 = Bundle By Name(cluster=w275, "5782 Trigger"="Trigger") -> (w274:T13)
          }
          event "Samples per 5782 record": Value Change {
            n168 = event-data() -> ()  [unwired: 1 in, 6 out]
            n169 = Unbundle By Name(w278) -> ("FPGA ref"=w281:T11)
            n170 = xnode "Read/Write Control"("FPGA VI Reference In"=w281, "5782 record length"="Samples per 5782 record") -> ("FPGA VI Reference Out"=w280:T11)  [unwired: 1 in, 1 out]
            n171 = Bundle By Name(cluster=w278, "FPGA ref"=w280, "samples per record"="Samples per 5782 record") -> (w277:T13)
          }
          event "Singleshot": Value Change {
            n172 = event-data() -> ()  [unwired: 1 in, 6 out]
            n173 = local write "Rumode"(FALSE ("Rumode")) -> ()
            n174 = Bundle By Name(cluster=w288, "scope mode"=ScopeMode."Single") -> (w283:T13)
            n175 = call "ToggleContinousMode.vi"("Cont Acquisition"=FALSE, "scope in"=w283) -> ("scope out"=w282:T13)  [unwired: 8 in, 1 out]
            n176 = call "ToggleAqcuisitionRunning_5782.vi"("Acquisition running"=TRUE, "scope in"=w282) -> ("scope out"=w286:T13)  [unwired: 8 in, 1 out]
            n177 = call "SendSWtrigger_5782.vi"("scope in"=w286) -> ("scope out"=w285:T13)  [unwired: 9 in, 1 out]
          }
          event "Rumode": Value Change {
            n178 = event-data() -> ()  [unwired: 1 in, 6 out]
            n179 = case shown="\"Triggered\"" "Trigmode" {
              tunnel: [ScopeMode."Running" ("scope mode") ScopeMode."Continuous" ("scope mode")] -> w291
              frame "Triggered" {
              }
              frame "Continuous" {
              }
            }
            n180 = Select(t=w291, s="Rumode", f=ScopeMode."Stopped" ("scope mode")) -> (s? t:f=w295:T14)
            n181 = Bundle By Name(cluster=w296, "scope mode"=w295) -> (w294:T13)
            n182 = case shown="\"Single\", \"Running\"" w295 {
              tunnel: w294 -> [w303 w310 w314]
              tunnel: [w304 w308 w315] -> w293
              frame "Single", "Running" {
                n183 = call "ToggleContinousMode.vi"("Cont Acquisition"=FALSE, "scope in"=w303) -> ("scope out"=w301:T13)  [unwired: 8 in, 1 out]
                n184 = call "ToggleAqcuisitionRunning_5782.vi"("Acquisition running"=TRUE, "scope in"=w301) -> ("scope out"=w305:T13)  [unwired: 8 in, 1 out]
                n185 = call "SendSWtrigger_5782.vi"("scope in"=w305) -> ("scope out"=w304:T13)  [unwired: 9 in, 1 out]
              }
              frame "Continuous" {
                n186 = call "ToggleAqcuisitionRunning_5782.vi"("Acquisition running"=TRUE, "scope in"=w310) -> ("scope out"=w309:T13)  [unwired: 8 in, 1 out]
                n187 = call "ToggleContinousMode.vi"("Cont Acquisition"=TRUE ("Acquisition running"), "scope in"=w309) -> ("scope out"=w308:T13)  [unwired: 8 in, 1 out]
              }
              frame "Stopped" {
                n188 = call "ToggleContinousMode.vi"("Cont Acquisition"=FALSE, "scope in"=w314) -> ("scope out"=w312:T13)  [unwired: 8 in, 1 out]
                n189 = call "ToggleAqcuisitionRunning_5782.vi"("Acquisition running"=FALSE, "scope in"=w312) -> ("scope out"=w315:T13)  [unwired: 8 in, 1 out]
              }
            }
          }
          event Value Change {
            n190 = event-data() -> ("CtlRef"=w319:refnum<vi>, "NewVal"=w317:bool)  [unwired: 1 in, 4 out]
            n191 = Search 1D Array(1D array=w320, element=w319) -> (index of element=w318:i32)  [unwired: 1 in]
            n192 = property on="Upper graph" class="WFGraph (strict)"("Active Plot"=w318, "Plot.Visible?"=w317) -> ()  [unwired: 2 in, 2 out]
            n193 = property on="Upper chart" class="WFChart (strict)"("Active Plot"=w318, "Plot.Visible?"=w317) -> ()  [unwired: 2 in, 2 out]
          }
          event Value Change {
            n194 = event-data() -> ("CtlRef"=w325:refnum<vi>, "NewVal"=w322:bool)  [unwired: 1 in, 4 out]
            n195 = Search 1D Array(1D array=w324, element=w325) -> (index of element=w323:i32)  [unwired: 1 in]
            n196 = property on="freqdata" class="WFGraph (strict)"("Active Plot"=w323, "Plot.Visible?"=w322) -> ()  [unwired: 2 in, 2 out]
            n197 = property on="Lower chart" class="WFChart (strict)"("Active Plot"=w323, "Plot.Visible?"=w322) -> ()  [unwired: 2 in, 2 out]
          }
          event "stop": Value Change {
            n198 = event-data() -> ()  [unwired: 1 in, 6 out]
          }
          event Value Change {
            n199 = event-data() -> ()  [unwired: 1 in, 6 out]
            n200 = case shown="\"V\"" "Unit" {
              tunnel: ["V" "dBV" "V^2"] -> w331
              frame "V" {
              }
              frame "dBV" {
              }
              frame "V^2" {
              }
            }
            n201 = Concatenate Strings("Amplitude [", w331, "]") -> (w329:string)
            n202 = property on="freqdata" class="WFGraph (strict)"("YScale.NameLbl.Text"=w329) -> ()  [unwired: 2 in, 2 out]
          }
          event "#bins": Value Change {
            n203 = event-data() -> ()  [unwired: 1 in, 6 out]
            n204 = local read "Upper chart"() -> (w340:dbl[][])
            n205 = local read "Window"() -> (w341:T8)
            n206 = local read "Unit"() -> (w342:T7)
            n207 = call "calc FFT.vi"("#bins"="#bins", "dt"=1e-06, "Unit"=w342, "Window"=w341, "data"=w340) -> ("Power Spectrum / PSD"=w339:cluster{"f0":dbl, "df":dbl, "magnitude":dbl[]}[])  [unwired: 6 in]
            n208 = local write "freqdata"(w339) -> ()
          }
          event "Zoom time X", "Zoom time Y": Value Change {
            n209 = event-data() -> ()  [unwired: 1 in, 6 out]
            n210 = control-ref of="Upper chart"() -> (w347:refnum<vi>)
            n211 = control-ref of="Upper graph"() -> (w348:refnum<vi>)
            n212 = call "setZoomTool.vi"("Zoom Y"="Zoom time Y", "Zoom  X"="Zoom time X", "reference"=w347) -> ()  [unwired: 9 in]
            n213 = call "setZoomTool.vi"("Zoom Y"="Zoom time Y", "Zoom  X"="Zoom time X", "reference"=w348) -> ()  [unwired: 9 in]
          }
          event "Zoom freq Y", "Zoom freq X": Value Change {
            n214 = event-data() -> ()  [unwired: 1 in, 6 out]
            n215 = control-ref of="Lower chart"() -> (w353:refnum<vi>)
            n216 = control-ref of="Lower graph"() -> (w352:refnum<vi>)
            n217 = control-ref of="freqdata"() -> (w354:refnum<vi>)
            n218 = call "setZoomTool.vi"("Zoom Y"="Zoom freq Y", "Zoom  X"="Zoom freq X", "reference"=w354) -> ()  [unwired: 9 in]
            n219 = call "setZoomTool.vi"("Zoom Y"="Zoom freq Y", "Zoom  X"="Zoom freq X", "reference"=w353) -> ()  [unwired: 9 in]
            n220 = call "setZoomTool.vi"("Zoom Y"="Zoom freq Y", "Zoom  X"="Zoom freq X", "reference"=w352) -> ()  [unwired: 9 in]
          }
          event Value Change {
            w358 = dbl[][] [] ("History Data")
            n221 = event-data() -> ()  [unwired: 1 in, 6 out]
            n222 = property on="Upper chart" class="WFChart (strict)"("History Data"=w358) -> ()  [unwired: 2 in, 2 out]
            n223 = property on="Lower chart" class="WFChart (strict)"("History Data"=w358) -> ()  [unwired: 2 in, 2 out]
            n224 = local write "freqdata"(cluster{"f0":dbl, "df":dbl, "magnitude":dbl[]}[] [] ("freqdata")) -> ()
            n225 = call "UpdateGraphs.vi"("Buffer mode"="Buffer", "Display mode"="Display", "Graph_refs"=w359) -> ()  [unwired: 9 in]
            n226 = property on="Zoom time X" class="Bool (strict)"("Val(Sgnl)"=TRUE ("Value (Signaling)")) -> ()  [unwired: 2 in, 2 out]
          }
        }
      }
      "stop 2" <- w94
    }
    frame Error {
    }
  }
  n227 = Unregister For Events(event registration refnum=w53) -> ()  [unwired: 1 in, 1 out]
  n228 = Unbundle By Name(w32) -> ("FPGA ref"=w61:T11)
  n229 = xnode "Close FPGA VI Reference"("FPGA VI Reference In"=w61) -> ()  [unwired: 1 in, 1 out]
